vi "writeToXML.vi"(8 "error in (no error)":errorcluster, 10 "ClassLabel":string, 11 "ClearCollOffset in":refnum<class "ClearCollOffset.lvclass">) -> (0 "error out":errorcluster, 2 "XML out":string, 3 "ClearCollOffset out":refnum<class "ClearCollOffset.lvclass">)   [LabVIEW 2014, in "TCSDataDefinitions.lvlib" / "TCSCommand.lvlib" / "OffsetCommands.lvlib" / "ClearCollOffset.lvclass"]
uses:
  ClearCollOffset.lvclass
  CollimationOffsetCommands/CollimationOffsetCommands.lvclass
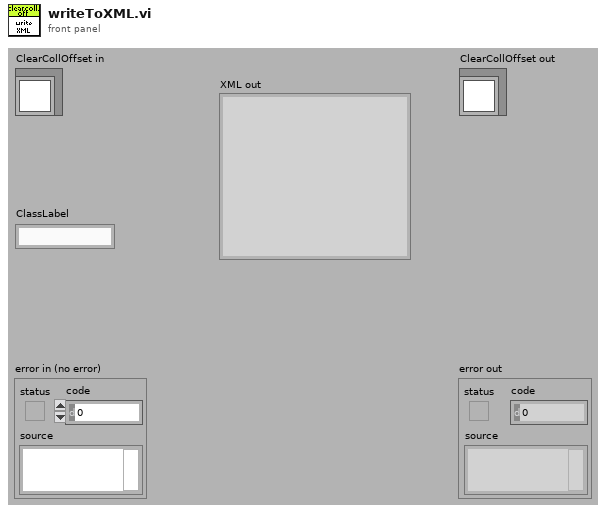
[diagram p1: front panel]
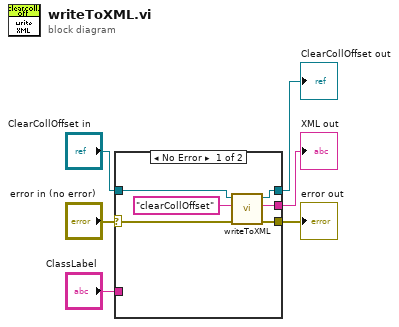
[diagram p0: block diagram]
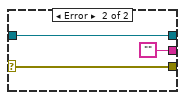
[diagram p2: hidden frame]
diagram:
  n1 = case shown="No Error" "error in (no error)" {
    selector: "error in (no error)" -> [w12 w15]
    tunnel: [w11 w15] -> w5
    tunnel: [w9 w14] -> w3
    tunnel: "ClearCollOffset in" -> [w10 w14]
    tunnel: [w8 ""] -> w2
    tunnel: "ClassLabel" -> [_ _]
    frame No Error {
      n2 = call-parent "writeToXML.vi"("error in (no error)"=w12, "ClassLabel"="clearCollOffset", "CollimationOffsetCommands in"=w10) -> ("error out"=w11:errorcluster, "XML out"=w8:string, "CollimationOffsetCommands out"=w9:refnum<class "ClearCollOffset.lvclass">)  [unwired: 6 in]
    }
    frame Error {
    }
  }
  "error out" <- w5
  "ClearCollOffset out" <- w3
  "XML out" <- w2
